vi "Auton.vi"(11 "Auton Array":dbl[][](array[numeric])) -> ()   [LabVIEW 2016]
uses:
  TestBench/Robot Global Data.vi
panel:
  out "Drive Speed":dbl
  out "Time Left":dbl
  in  "Action Variables":enum32{"Idle - 0", "Driving - 2", "Turning - 2"}(tab)
  out "Turn Error":dbl
  in  "Angle Threshold":dbl=1.0
  in  "Max Turn Speed":dbl=0.7
  in  "kI":dbl=0.00025
  in  "kP":dbl=0.008
  out "Turn Speed":dbl
  out "Integral Value":dbl
  out "Step Start Time":u32
  out "Step":i32
  # "Local Variables"
  # "Auton CSV (tab) Format -\n\n(Action)\\t      (Setpoint)\\t       (Timeout)\\t        (Var 1)\\t         (Var 2)\\t         (Var 3)\\t\n\n2       90       10000       0       0       0"
  # "Turning PI Control"
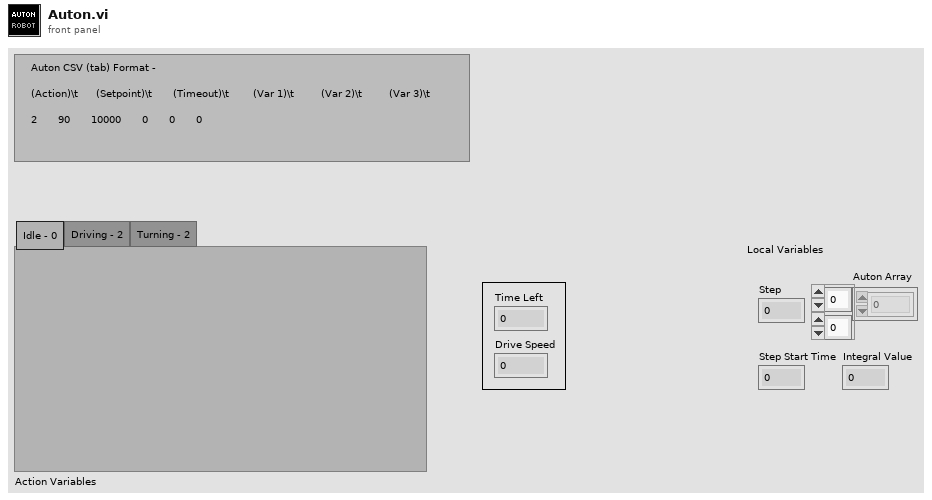
[diagram p1: front panel]
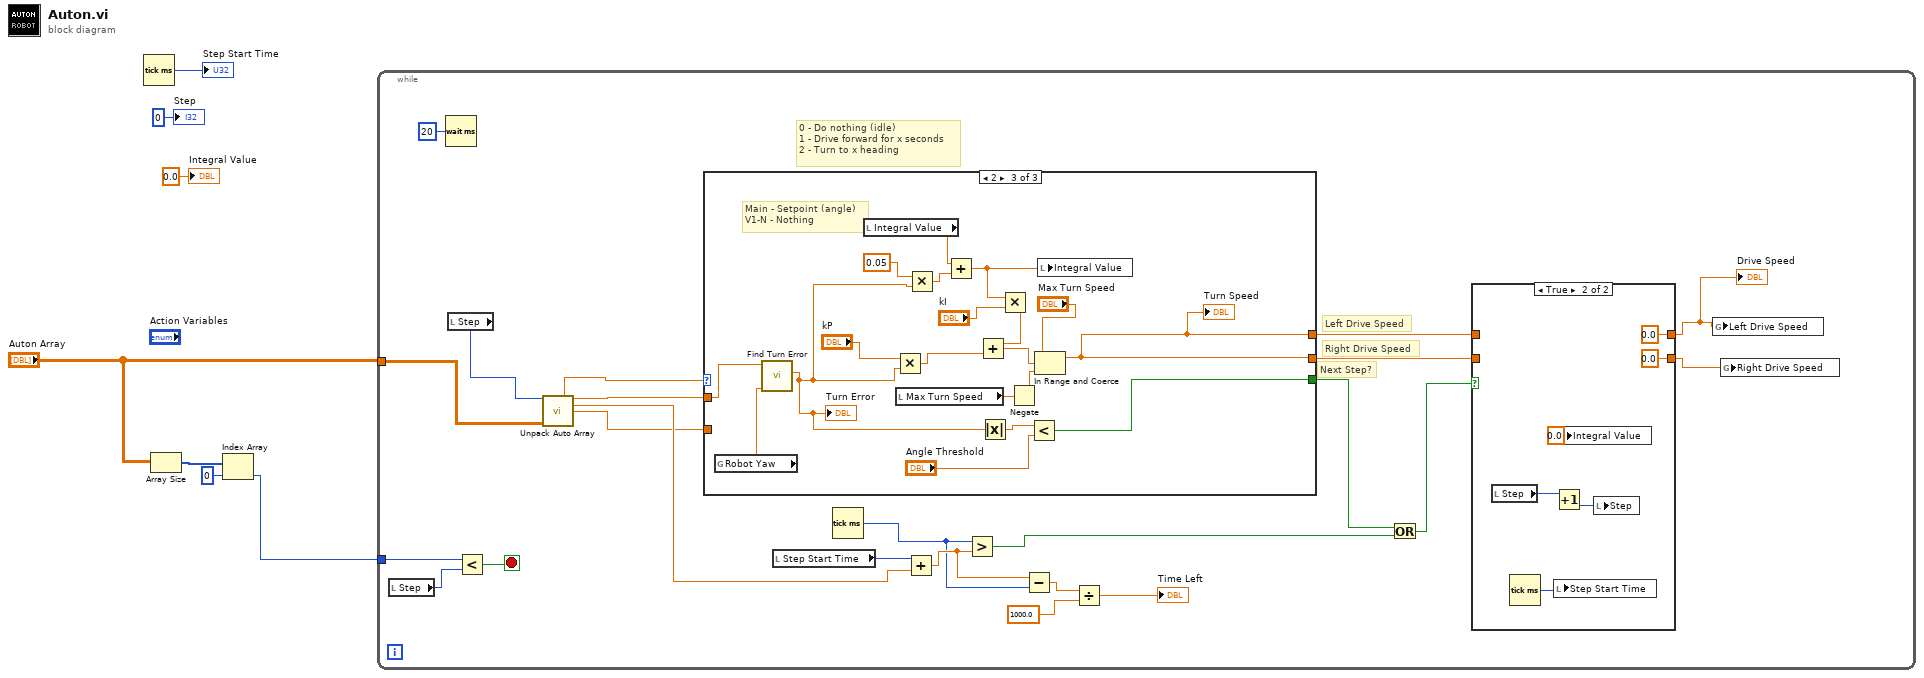
[diagram p0: block diagram]
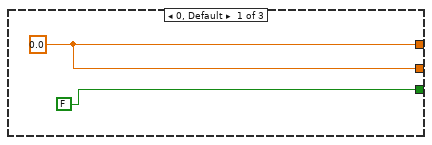
[diagram p3: hidden frame]
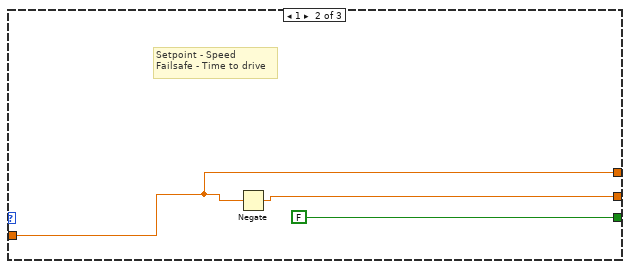
[diagram p4: hidden frame]
diagram:
  n1 = Tick Count (ms)() -> (millisecond timer value=→"Step Start Time":u32)
  n2 = Array Size(array="Auton Array") -> (size(s)=w5:i32[])
  n3 = Index Array(array=w5, index=0) -> (element=w3:i32)
  n4 = while {
    tunnel: "Auton Array" -> [w19]
    tunnel: w3 -> [w24]
    stop <- w23 stop-if-true
    # "Next Step?"
    # "Right Drive Speed"
    # "Left Drive Speed"
    # "0 - Do nothing (idle)\n1 - Drive forward for x seconds\n2 - Turn to x heading"
    n5 = local read "Step"() -> (w25:i32)
    n6 = Wait (ms)(milliseconds to wait=u32 20) -> ()  [unwired: 1 out]
    n7 = local read "Step"() -> (w20:i32)
    n8 = Less?(x=w24, y=w25) -> (x < y?=w23:bool)
    n9 = call "Unpack Auto Array.vi"("Step"=w20, "Auton Array"=w19) -> ("Action Type"=w18:dbl, "Setpoint"=w17:dbl, "Time Failsafe"=w16:dbl, "Var 1"=w15:dbl)  [unwired: 8 in, 2 out]
    n10 = case shown="2" w18 {
      tunnel: [FALSE FALSE w61] -> w28
      tunnel: w15 -> [_ _ _]
      tunnel: [w39 w41 w47] -> w14
      tunnel: [w39 w42 w47] -> w22
      tunnel: w17 -> [_ w41 w46]
      frame 0, Default {
        w39 = 0.0 ("Numeric")
      }
      frame 1 {
        # "Setpoint - Speed\nFailsafe - Time to drive"
        n11 = Negate(x=w41) -> (-x=w42:dbl)
      }
      frame 2 {
        # "Main - Setpoint (angle)\nV1-N - Nothing"
        n12 = global read "Robot Global Data.vi" "Robot Yaw"() -> (w45:dbl)
        n13 = call "Find Turn Error.vi"("Target Angle"=w46, "Current Angle"=w45) -> ("Error"=w44:dbl)  [unwired: 7 in]
        "Turn Error" <- w44
        n14 = local read "Integral Value"() -> (w56:dbl)
        n15 = Multiply(x="kP", y=w44) -> (x*y=w58:dbl)
        n16 = local read "Max Turn Speed"() -> (w50:dbl)
        n17 = Multiply(x=0.05, y=w44) -> (x*y=w59:dbl)
        n18 = Add(x=w56, y=w59) -> (x+y=w54:dbl)
        n19 = Absolute Value(x=w44) -> (abs(x)=w62:dbl)
        n20 = Multiply(x=w54, y="kI") -> (x*y=w55:dbl)
        n21 = Add(x=w55, y=w58) -> (x+y=w57:dbl)
        n22 = Negate(x=w50) -> (-x=w49:dbl)
        n23 = Less?(x=w62, y="Angle Threshold") -> (x < y?=w61:bool)
        n24 = In Range and Coerce(upper limit="Max Turn Speed", x=w57, lower limit=w49) -> (coerced(x)=w47:dbl)  [unwired: 1 out]
        "Turn Speed" <- w47
        n25 = local write "Integral Value"(w54) -> ()
      }
    }
    n26 = local read "Step Start Time"() -> (w29:u32)
    n27 = Tick Count (ms)() -> (millisecond timer value=w12:u32)
    n28 = Add(x=w29, y=w16) -> (x+y=w13:dbl)
    n29 = Greater?(x=w12, y=w13) -> (0:w27:bool)
    n30 = Subtract(x=w13, y=w12) -> (x-y=w11:dbl)
    n31 = Divide(x=w11, y=1000.0) -> (x/y=→"Time Left":dbl)
    n32 = Or(x=w28, y=w27) -> (x .or. y?=w26:bool)
    n33 = case shown="True" w26 {
      tunnel: [w32 0.0 ("output")] -> w8
      tunnel: w14 -> [w32 _]
      tunnel: [w31 0.0 ("output")] -> w21
      tunnel: w22 -> [w31 _]
      frame False {
      }
      frame True {
        n34 = local read "Step"() -> (w37:i32)
        n35 = Tick Count (ms)() -> (millisecond timer value=w38:u32)
        n36 = Increment(x=w37) -> (x+1=w36:i32)
        n37 = local write "Step Start Time"(w38) -> ()
        n38 = local write "Integral Value"(0.0 ("Integral")) -> ()
        n39 = local write "Step"(w36) -> ()
      }
    }
    "Drive Speed" <- w8
    n40 = global write "Robot Global Data.vi" "Left Drive Speed"(w8) -> ()
    n41 = global write "Robot Global Data.vi" "Right Drive Speed"(w21) -> ()
  }
  "Step" <- i8 0 ("Step")
  "Integral Value" <- 0.0 ("Integral")
